vi "Periodic Log Filter Check2.vi"(5 "Remove Immediately?(F)":bool, 6 "Exceeding processing capacity(F)":bool, 7 "reset?":bool, 8 "Settings":T4={"threashold(#/s)"=2.0, "Check Peroid(s)"=1.0}, 11 "Cross CSM Data":T1={"Name(\"\" to use uuid)"="CSM Tiny", "Current State"="UI: Refresh Buttons", "Arguments"="", "Source Message"={"‘State"="", "’Arguments"="", "’Error"={"status"=FALSE, "code"=0, "source"=""}}, "Source Module"="<end>", "Complete(T)/Start(F)"=TRUE, "LogType"=enum."State Change", "Time Stamp"=timestamp(0 s since 1904-01-01)}) -> (0 "Filtered":bool, 1 "additional Info":string[](array[string]), 2 "current time":timestamp, 3 "Cross CSM Data out":T1={"Name(\"\" to use uuid)"="", "Current State"="", "Arguments"="", "Source Message"={"‘State"="", "’Arguments"="", "’Error"={"status"=FALSE, "code"=0, "source"=""}}, "Source Module"="", "Complete(T)/Start(F)"=FALSE, "LogType"=enum."State Change", "Time Stamp"=timestamp(0 s since 1904-01-01)}, 4 "Filtered Status":string[](array[string]))   [LabVIEW 2017, in "Communicable State Machine.lvlib" / "LogFilter.lvclass"]
uses:
  LogFilter.lvclass
  Typedef/_CSM_GlobalLog_MSG.ctl
  Typedef/_CSM_Response Source Message.ctl
  Typedef/_CSM_GlobalLog_MSG_TYPE.ctl
  Utility/Periodic String Filter State.ctl
  Communicable State Machine.lvlib
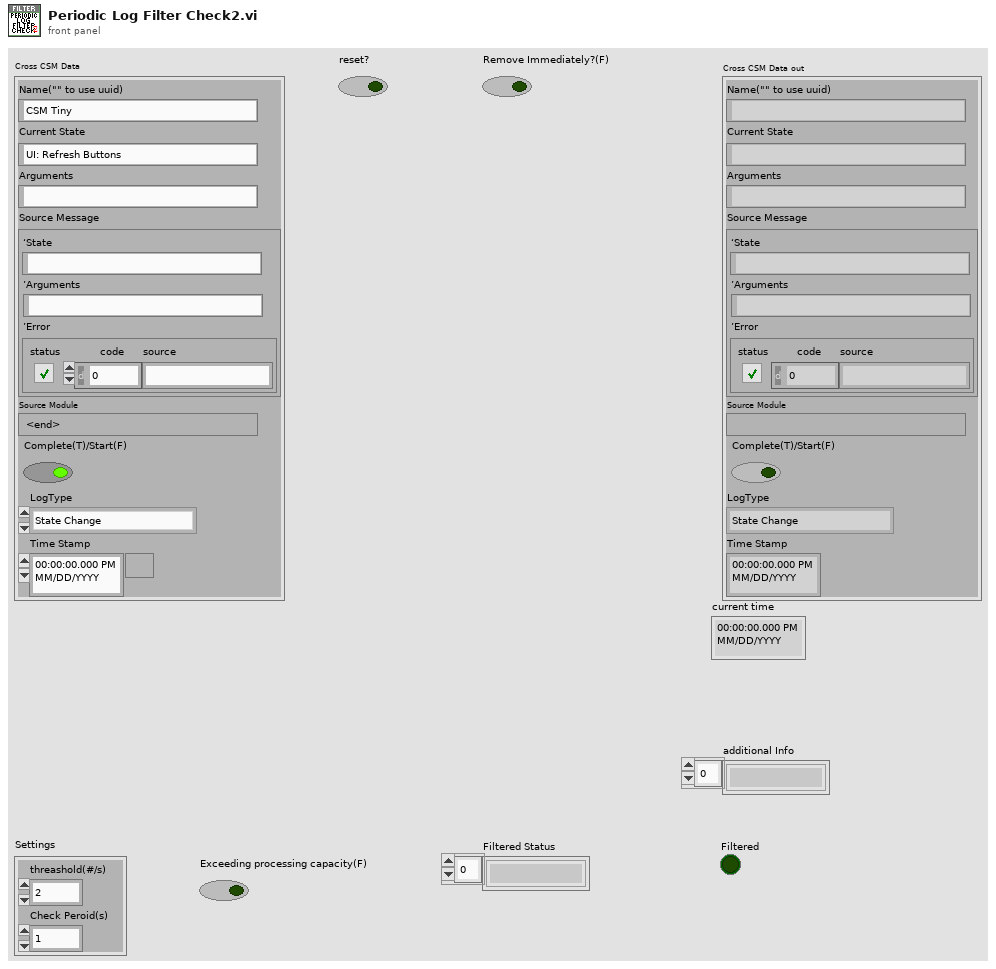
[diagram p1: front panel]
types:
  T1 = typedef "Communicable State Machine.lvlib/_CSM_GlobalLog_MSG.ctl" = cluster{"Name(\"\" to use uuid)":string, "Current State":string, "Arguments":string, "Source Message":T2, "Source Module":string, "Complete(T)/Start(F)":bool, "LogType":T3, "Time Stamp":timestamp}
  T2 = typedef "Communicable State Machine.lvlib/_CSM_Response Source Message.ctl" = cluster{"‘State":string, "’Arguments":string, "’Error":errorcluster}
  T3 = typedef "Communicable State Machine.lvlib/_CSM_GlobalLog_MSG_TYPE.ctl" = enum16{"User Log", "State Change", "Status", "Interrupt", "Register", "Unregister", "Error Log", "Module Created", "Module Destroyed"}
  T4 = cluster{"threashold(#/s)":dbl, "Check Peroid(s)":dbl}
  T5 = typedef "Communicable State Machine.lvlib/Periodic String Filter State.ctl" = enum16{"Normal", "Remove All Filters"}
  T6 = typedef "Communicable State Machine.lvlib/Periodic String Filter Info.ctl" = cluster{"String":string, "Count":i64, "since":timestamp, "param":string}
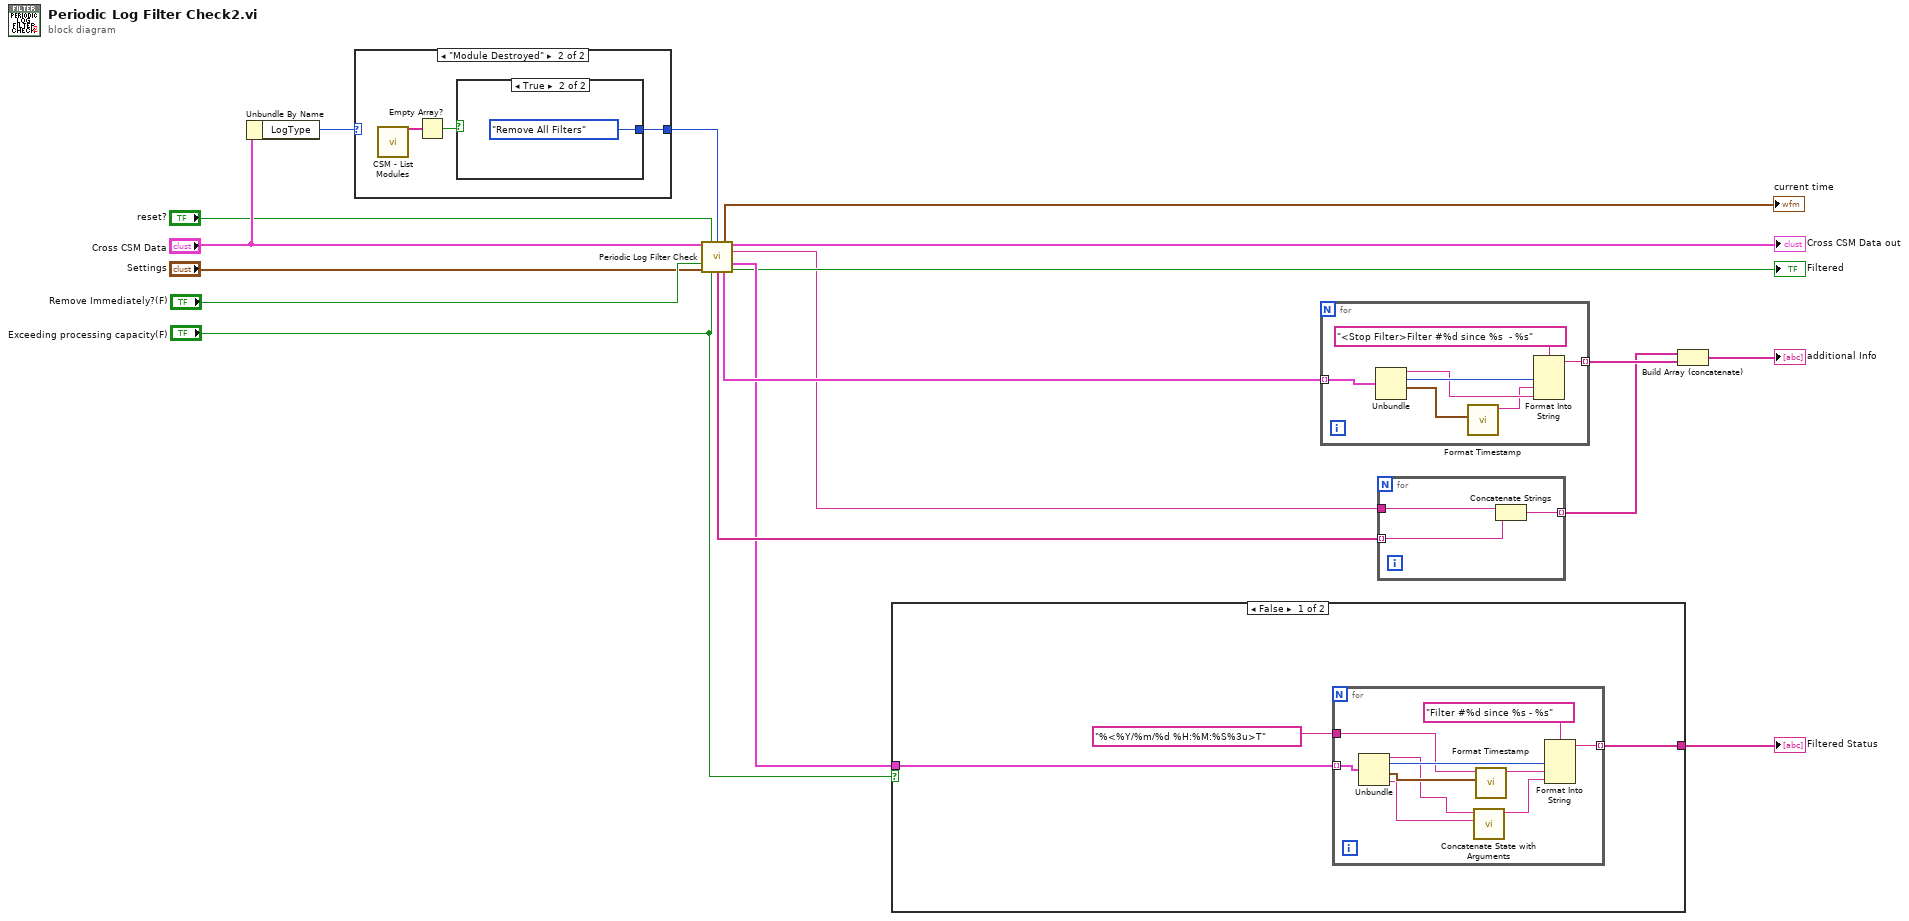
[diagram p0: block diagram]
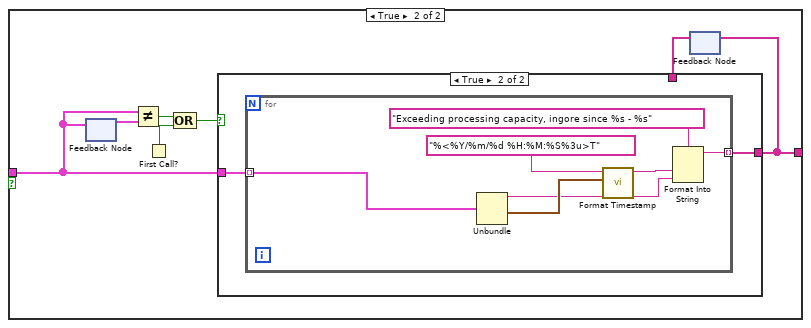
[diagram p2: hidden frame]
diagram:
  n1 = Unbundle By Name("Cross CSM Data") -> ("LogType"=w8:T3)
  n2 = case shown="\"Module Destroyed\"" w8 {
    tunnel: [_ w19] -> w7
    frame "User Log", Default {
    }
    frame "Module Destroyed" {
      n3 = call "CSM - List Modules.vi"() -> ("Module Names"=w21:string[])  [unwired: 10 in, 1 out]
      n4 = Empty Array?(array=w21) -> (empty?=w20:bool)
      n5 = case shown="True" w20 {
        tunnel: [_ Periodic_String_Filter_State."Remove All Filters" ("State")] -> w19
        frame False {
        }
        frame True {
        }
      }
    }
  }
  n6 = call "Periodic Log Filter Check.vi"("Cross CSM Data"="Cross CSM Data", "reset?"="reset?", "State"=w7, "Remove Immediately?(F)"="Remove Immediately?(F)", "Settings"="Settings", "Exceeding processing capacity(F)"="Exceeding processing capacity(F)") -> ("current time"=→"current time":timestamp, "Cross CSM Data out"=→"Cross CSM Data out":T1, "oper"=w2:string, "Filtered Status"=w12:T6[], "added Info"=w18:string[], "removed info"=w17:T6[], "Filtered"=→"Filtered":bool)  [unwired: 3 in]
  n7 = case shown="False" "Exceeding processing capacity(F)" {
    tunnel: w12 -> [w25 w37]
    tunnel: [w24 w42] -> w5
    frame False {
      n8 = for {
        tunnel: w25 -> [w34] mode=indexing
        tunnel: [w35] -> w24 mode=indexing
        tunnel: "%<%Y/%m/%d %H:%M:%S%3u>T" ("format string") -> [w27]
        n9 = Unbundle(w34) -> ("String"=w29:string, "Count"=w33:i64, "since"=w31:timestamp, "param"=w26:string)
        n10 = call "Concatenate State with Arguments.vi"("Arguments"=w26, "State"=w29) -> ("State with Arguements"=w28:string)  [unwired: 9 in]
        n11 = call "Format Timestamp.vi"("timestamp"=w31, "format string"=w27) -> ("String"=w30:string)  [unwired: 9 in]
        n12 = Format Into String(format string="Filter #%d since %s - %s", w33, w30, w28) -> (resulting string=w35:string)  [unwired: 2 in, 1 out]
      }
    }
    frame True {
      n13 = feedback #1() -> (w38:T6[])  [unwired: 1 in]
      n14 = feedback-in #1(w37) -> ()
      n15 = Not Equal?(x=w37, y=w38) -> (x != y?=w39:bool)
      n16 = First Call?() -> (First Call?: T/F=w40:bool)
      n17 = Compound Arithmetic op=OR(w39, w40) -> (w36:bool)
      n18 = feedback #2() -> (w41:string[])  [unwired: 1 in]
      n19 = case shown="True" w36 {
        tunnel: [w43 w45] -> w42
        tunnel: w37 -> [_ w44]
        tunnel: w41 -> [w43 _]
        frame False {
        }
        frame True {
          n20 = for {
            tunnel: w44 -> [w51] mode=indexing
            tunnel: [w52] -> w45 mode=indexing
            n21 = Unbundle(w51) -> ("String"=w47:string, "since"=w49:timestamp)  [unwired: 2 out]
            n22 = call "Format Timestamp.vi"("timestamp"=w49, "format string"="%<%Y/%m/%d %H:%M:%S%3u>T") -> ("String"=w48:string)  [unwired: 9 in]
            n23 = Format Into String(format string="Exceeding processing capacity, ingore since %s - %s", w48, w47) -> (resulting string=w52:string)  [unwired: 2 in, 1 out]
          }
        }
      }
      n24 = feedback-in #2(w42) -> ()
    }
  }
  "Filtered Status" <- w5
  n25 = for {
    tunnel: w17 -> [w54] mode=indexing
    tunnel: [w53] -> w16 mode=indexing
    n26 = Unbundle(w54) -> ("String"=w57:string, "Count"=w58:i64, "since"=w56:timestamp)  [unwired: 1 out]
    n27 = call "Format Timestamp.vi"("timestamp"=w56) -> ("String"=w55:string)  [unwired: 10 in]
    n28 = Format Into String(format string="<Stop Filter>Filter #%d since %s  - %s", w58, w55, w57) -> (resulting string=w53:string)  [unwired: 2 in, 1 out]
  }
  n29 = for {
    tunnel: w18 -> [w62] mode=indexing
    tunnel: [w61] -> w15 mode=indexing
    tunnel: w2 -> [w60]
    n30 = Concatenate Strings(w60, w62) -> (w61:string)
  }
  n31 = Build Array (concatenate)(w15, w16) -> (→"additional Info":string[])
